vi "Conveyer Belt Global Data.vi"() -> ()   [LabVIEW 2012]
panel:
  in  "Conveyer Belt Information":T1
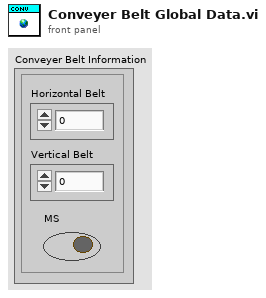
[diagram p1: front panel]
types:
  T1 = cluster{"Horizontal Belt":dbl, "Vertical Belt":dbl, "MS":bool}
diagram:
